vi "IndexMatching.vi"(1 "Array2":i32[](array[numeric])=[1, 2, 3, 4], 2 "Array1":i32[](array[numeric])=[0, 4, 7, 2]) -> (0 "Matched Indices":i32[](array[numeric]))   [LabVIEW 2010]
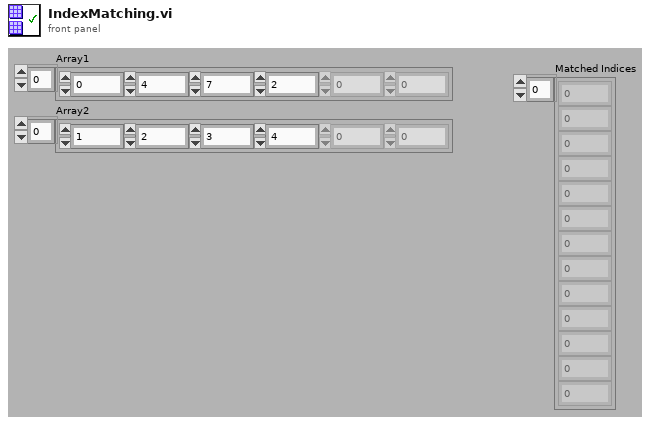
[diagram p1: front panel]
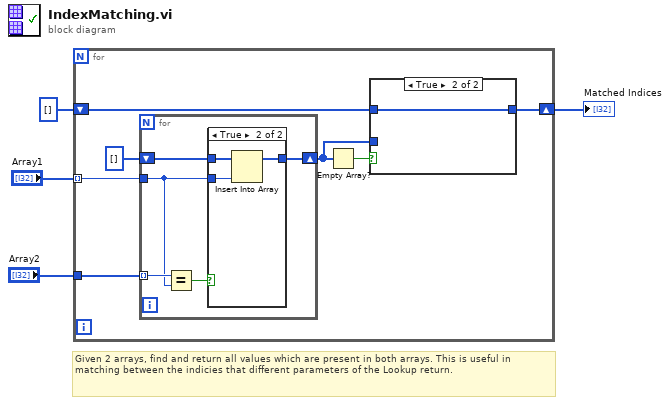
[diagram p0: block diagram]
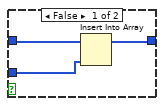
[diagram p2: hidden frame]
diagram:
  # "Given 2 arrays, find and return all values which are present in both arrays. This is useful in matching between the indicies that different parameters of the Lookup return."
  n1 = for {
    tunnel: "Array1" -> [w10] mode=indexing
    tunnel: "Array2" -> [w11]
    shift-right: [w6] -> w1
    shift-left: i32[] [] -> [w7]
    n2 = for {
      tunnel: w11 -> [w18] mode=indexing
      tunnel: w10 -> [w17]
      shift-right: [w16] -> w5
      shift-left: i32[] [] -> [w19]
      n3 = Equal?(x=w18, y=w17) -> (x = y?=w20:bool)
      n4 = case shown="True" w20 {
        tunnel: w19 -> [w21 w24]
        tunnel: w17 -> [_ w23]
        tunnel: [w21 w22] -> w16
        frame False {
        }
        frame True {
          n5 = Insert Into Array(array=w24, new element=w23) -> (w22:i32[])  [unwired: 1 in]
        }
      }
    }
    n6 = Empty Array?(array=w5) -> (empty?=w8:bool)
    n7 = case shown="True" w8 {
      tunnel: w7 -> [w14 w15]
      tunnel: [w12 w15] -> w6
      tunnel: w5 -> [w13 _]
      frame False {
        n8 = Insert Into Array(array=w14, new element=w13) -> (w12:i32[])  [unwired: 1 in]
      }
      frame True {
      }
    }
  }
  "Matched Indices" <- w1
